vi "SaveFinalFile.vi"(7 "Sample name":string, 8 "error in (no error)":errorcluster, 9 "Type":string, 10 "Text":string, 11 "Path":path) -> (0 "error out":errorcluster)   [LabVIEW 2014]
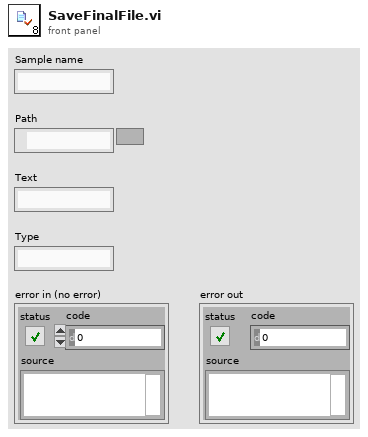
[diagram p1: front panel]
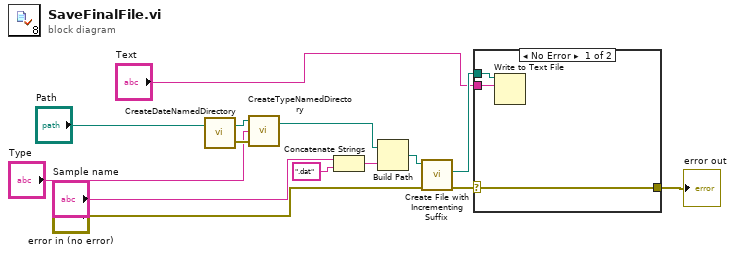
[diagram p0: block diagram]
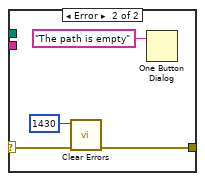
[diagram p2: hidden frame]
diagram:
  n1 = call "CreateDateNamedDirectory.vi"("base path"="Path") -> ("error out"=w11:errorcluster, "created path"=w12:path)  [unwired: 1 in]
  n2 = call "CreateTypeNamedDirectory.vi"("error in"=w11, "type"="Type", "base path"=w12) -> ("created path"=w9:path)  [unwired: 1 out]
  n3 = Concatenate Strings("Sample name", ".dat" ("string")) -> (w5:string)
  n4 = Build Path(base path=w9, name or relative path=w5) -> (appended path=w8:path)
  n5 = call <vilib>:"Create File with Incrementing Suffix.vi"("error in (no error)"="error in (no error)", "file path"=w8) -> ("error out"=w3:errorcluster, "actual path"=w14:path)  [unwired: 7 in, 1 out]
  n6 = case shown="No Error" w3 {
    selector: w3 -> [w15 w21]
    tunnel: w14 -> [w17 _]
    tunnel: "Text" -> [w16 _]
    tunnel: [w15 w20] -> w2
    frame No Error {
      n7 = Write to Text File(file (use dialog)=w17, text=w16) -> ()  [unwired: 2 in, 3 out]
    }
    frame Error {
      n8 = call <vilib>:"Clear Errors.vi"("error in (no error)"=w21, "specific error code to clear (0: all)"=1430) -> ("error out"=w20:errorcluster)  [unwired: 4 in, 1 out]
      n9 = One Button Dialog(message="The path is empty" ("error source (\" \")")) -> ()  [unwired: 1 in, 1 out]
    }
  }
  "error out" <- w2
